vi "XML Reader Init.vi"(8 "error in":errorcluster, 11 "File Path (dialog if empty)":path) -> (0 "error out":errorcluster, 3 "XML Reader out":T1)   [LabVIEW 2016, in "Pathloss XML Reader.lvlib"]
uses:
  Pathloss XML Reader.lvlib
  Controls/XML Reader Data Ref.ctl
  Controls/XML Reader Data.ctl
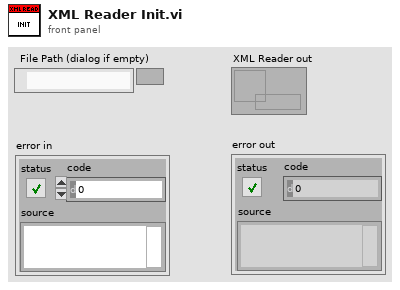
[diagram p1: front panel]
types:
  T1 = typedef "Pathloss XML Reader.lvlib/XML Reader Data Ref.ctl" = refnum<data-value>
  T2 = typedef "Pathloss XML Reader.lvlib/XML Reader Data.ctl" = cluster{"Remaining XML":string, "Section Name Stack":string[], "Section Stack":string[]}
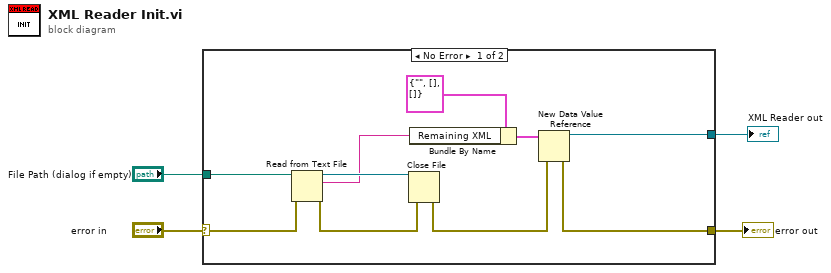
[diagram p0: block diagram]
diagram:
  n1 = case shown="No Error" "error in" {
    selector: "error in" -> [w13 w15]
    tunnel: "File Path (dialog if empty)" -> [w14 _]
    tunnel: [w6 w15] -> w2
    tunnel: [w5 _] -> w1
    frame No Error {
      n2 = Read from Text File(file (use dialog)=w14, error in=w13) -> (refnum out=w11:refnum<file>, text=w9:string, error out=w12:errorcluster)  [unwired: 2 in, 1 out]
      n3 = Close File(refnum=w11, error in=w12) -> (error out=w7:errorcluster)  [unwired: 1 out]
      n4 = Bundle By Name(cluster=T2 {"Remaining XML"="", "Section Name Stack"=[], "Section Stack"=[]} ("XML Reader State Element"), "Remaining XML"=w9) -> (w8:T2)
      n5 = New Data Value Reference(data value=w8, error in=w7) -> (data value reference=w5:refnum<data-value>, error out=w6:errorcluster)
    }
    frame Error {
    }
  }
  "error out" <- w2
  "XML Reader out" <- w1
